vi "Ex3strip.vi"() -> ()   [LabVIEW 2010]
panel:
  out "Strip 3":sgl[](graph)
  out "Strip 2":sgl[](graph)
  out "Strip 1":sgl[](graph)
  in  "Temperature":dbl=-10.0 format="%.2f"
  in  "Exposure":dbl min=0.0 step=0.001 format="%.3f"
  in  "stop":bool
  out "error out":errorcluster
  in  "error in (no error)":errorcluster
  # "Ex3strip.vi - \n3 strip example"
  # "Description: This example collects 3 strips \nfrom a CCD camera system. These 3 strips \nare displayed on the 3 separate graphs. You \ncan set the exposure and the temperature. \nTo finish example press the stop button."
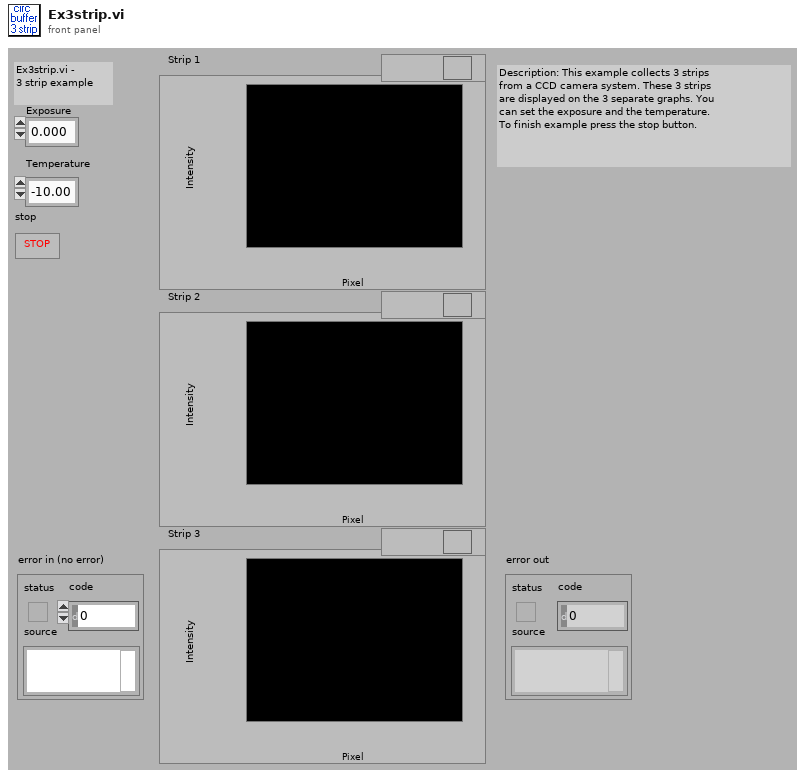
[diagram p1: front panel]
types:
  T1 = cluster{"Acquire focus mode,\nSync (circualar buffers)":i32, "Exposure":dbl, "Number of Images":i32, "Software Accumulation":i32}
  T2 = cluster{"Camera Handle":u32, "Pulser Handle":u32, "File Handle":u32, "Display Handle":u32, "Image Handle":u32}
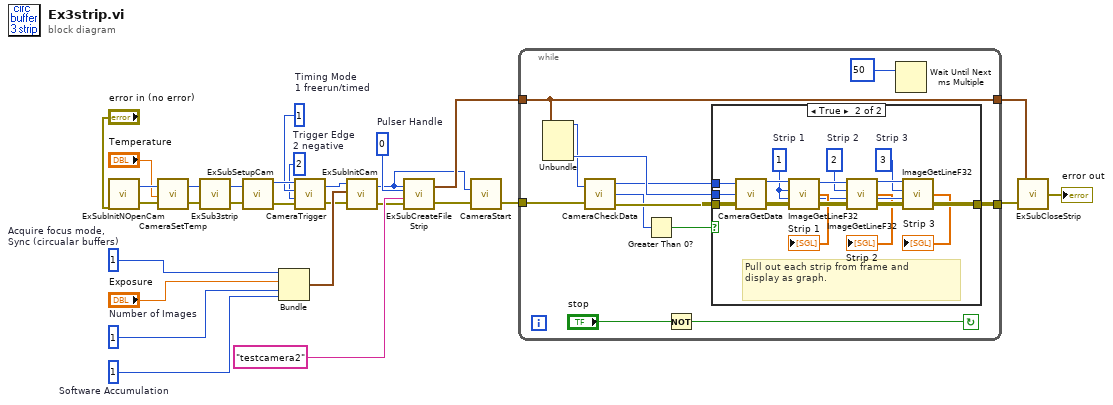
[diagram p0: block diagram]
diagram:
  w11 = 2  # Trigger Edge 2 negative
  w12 = 1  # Timing Mode 1 freerun/timed
  w21 = 0  # Pulser Handle
  w27 = 1  # Number of Images
  w28 = 1  # Acquire focus mode, Sync (circualar buffers)
  w26 = 1  # Software Accumulation
  n1 = call "ExSubInitNOpenCam.vi"("error in (no error)"="error in (no error)") -> ("Camera Handle"=w5:u32, "error out"=w6:errorcluster)
  n2 = call <userlib>:"CameraSetTemp.vi"("error in (no error)"=w6, "Temperature"="Temperature", "Camera Handle"=w5) -> ("error out"=w7:errorcluster, "Camera Handle"=w4:u32)
  n3 = call "ExSub3strip.vi"("error in (no error)"=w7, "Camera Handle"=w4) -> ("error out"=w3:errorcluster, "Camera Handle"=w2:u32)
  n4 = call "ExSubSetupCam.vi"("error in (no error)"=w3, "Camera Handle"=w2) -> ("error out"=w10:errorcluster, "Camera Handle"=w14:u32)
  n5 = Bundle("Acquire focus mode,\nSync (circualar buffers)"=w28, "Exposure"="Exposure", "Number of Images"=w27, "Software Accumulation"=w26) -> (w23:T1)  [unwired: 1 in]
  n6 = call <userlib>:"CameraTrigger.vi"("error in"=w10, "Trigger Edge"=w11, "Timing Mode"=w12, "Camera Handle"=w14) -> ("error out"=w15:errorcluster, "Camera Handle"=w13:u32)
  n7 = call "ExSubInitCam.vi"("error in (no error)"=w15, "Camera Information"=w23, "Camera Handle"=w13) -> ("error out"=w22:errorcluster, "Camera Handle"=w19:u32)
  n8 = call "ExSubCreateFileStrip.vi"("error in (no error)"=w22, "File and Display Name"="testcamera2", "Pulser Handle"=w21, "Camera Handle"=w19) -> ("error out"=w8:errorcluster, "Handles Out"=w20:T2)
  n9 = call <userlib>:"CameraStart.vi"("error in"=w8, "Camera Handle"=w19) -> ("error out"=w9:errorcluster)  [unwired: 1 out]
  n10 = while {
    tunnel: w20 -> [w38]
    tunnel: w9 -> [w37]
    tunnel: [w35] -> w17
    tunnel: [w38] -> w18
    stop <- w39 continue-if-true
    n11 = Unbundle(w38) -> ("Camera Handle"=w33:u32, "Image Handle"=w34:u32)  [unwired: 3 out]
    n12 = call <userlib>:"CameraCheckData.vi"("Camera Handle"=w33, "error in"=w37) -> ("Camera Handle"=w32:u32, "Number Of Frames Available"=w30:i32, "error out"=w36:errorcluster)
    n13 = Greater Than 0?(x=w30) -> (x > 0?=w31:bool)
    n14 = Not(x="stop") -> (.not. x?=w39:bool)
    n15 = case shown="True" w31 {
      tunnel: w36 -> [w42 w57]
      tunnel: [w42 w50] -> w35
      tunnel: w34 -> [_ w54]
      tunnel: w32 -> [_ w53]
      frame False {
      }
      frame True {
        w46 = 3  # Strip 3
        w43 = 2  # Strip 2
        w49 = 1  # Strip 1
        # "Pull out each strip from frame and\ndisplay as graph."
        n16 = call <userlib>:"CameraGetData.vi"("error in"=w57, "Data Handle"=w54, "Camera Handle"=w53) -> ("error out"=w56:errorcluster, "Data Handle"=w55:u32)  [unwired: 1 out]
        n17 = call <userlib>:"ImageGetLineF32.vi"("error in"=w56, "Z Position"=w49, "Y Position"=w49, "Data Handle"=w55) -> ("error out"=w52:errorcluster, "Array F32"=→"Strip 1":sgl[], "Data Handle"=w48:u32)
        n18 = call <userlib>:"ImageGetLineF32.vi"("error in"=w52, "Z Position"=w49, "Y Position"=w43, "Data Handle"=w48) -> ("error out"=w51:errorcluster, "Array F32"=→"Strip 2":sgl[], "Data Handle"=w47:u32)
        n19 = call <userlib>:"ImageGetLineF32.vi"("error in"=w51, "Z Position"=w49, "Y Position"=w46, "Data Handle"=w47) -> ("error out"=w50:errorcluster, "Array F32"=→"Strip 3":sgl[])  [unwired: 1 out]
      }
    }
    n20 = Wait Until Next ms Multiple(millisecond multiple=50) -> ()  [unwired: 1 out]
  }
  n21 = call "ExSubCloseStrip.vi"("error in (no error)"=w17, "Handles In"=w18) -> ("error out"=→"error out":errorcluster)
